vi "auxtesting_readMeasurementsCrossed.vi"() -> ()   [LabVIEW 2015, in "Tausand AB1000.lvlib"]
uses:
  <instrlib>/Tausand AB1000/Tausand AB1000.lvlib
  <instrlib>/Tausand AB1000/Public/Controls/deviceTypeRing.ctl
  <instrlib>/Tausand AB1000/Public/Controls/channelRing.ctl
panel:
  out "reading timer (s)":dbl
  out "error out":errorcluster
  in  "VISA resource name":refnum<visa-resource-name>
  in  "error in (no error)":errorcluster
  out "checksum ok?":bool
  out "read time":timestamp
  out "labels":string[](array[string])
  out "values":u32[](array[numeric])
  in  "channel":T1=1 items=["none", "A", "B", "C", "D", "E", "F", "G", "H"]
  in  "read timeout (500 ms)":u32=500
  in  "device type":T2 items=["any"=0, "AB1002"=1002, "AB1004"=1004, "AB1502"=1502, "AB1504"=1504, "AB1902"=1902, "AB1904"=1904, "AB2002"=2002, "AB2004"=2004, "AB2502"=2502, "AB2504"=2504, "AB2902"=2902, "AB2904"=2904]
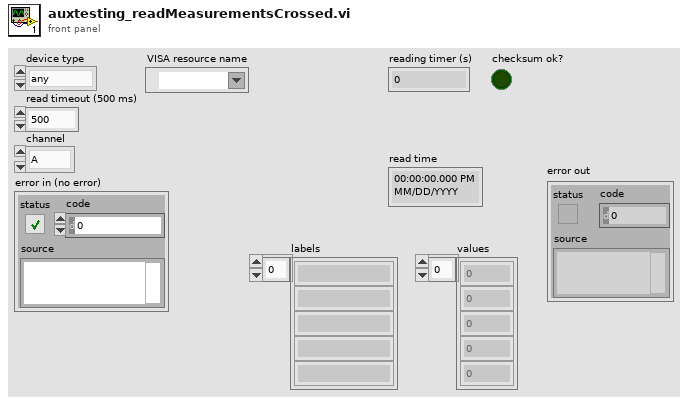
[diagram p1: front panel]
types:
  T1 = typedef "Tausand AB1000.lvlib/channelRing.ctl" = u8
  T2 = typedef "Tausand AB1000.lvlib/deviceTypeRing.ctl" = u16
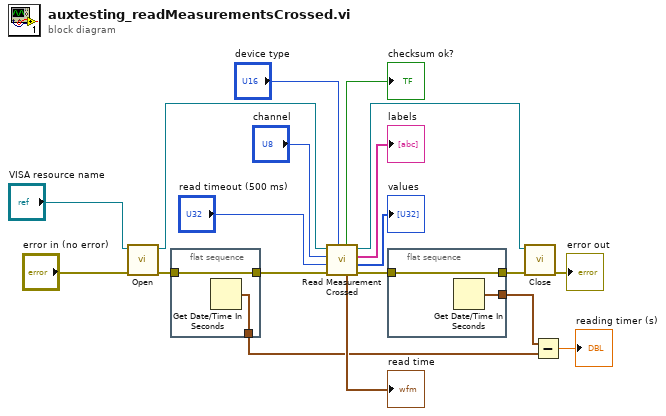
[diagram p0: block diagram]
diagram:
  n1 = call <instrlib>:"Open.vi"("error in (no error)"="error in (no error)", "VISA resource name"="VISA resource name") -> ("error out"=w6:errorcluster, "VISA resource name out"=w19:refnum<visa-resource-name>)  [unwired: 8 in]
  n2 = flat-sequence {
    tunnel: [w21] -> w7
    tunnel: w6 -> [w21]
    tunnel: [w20] -> w2
    frame #0 {
      n3 = Get Date/Time In Seconds() -> (seconds since 1Jan1904=w20:timestamp)
    }
  }
  n4 = call <instrlib>:"Read Measurement Crossed.vi"("device type"="device type", "error in (no error)"=w7, "read timeout (500 ms)"="read timeout (500 ms)", "channel"="channel", "VISA Refnum in"=w19) -> ("error out"=w5:errorcluster, "values"=→"values":u32[], "labels"=→"labels":string[], "VISA Refnum out"=w18:refnum<visa-resource-name>, "read time"=→"read time":timestamp, "checksum ok?"=→"checksum ok?":bool)  [unwired: 1 in]
  n5 = flat-sequence {
    tunnel: [w23] -> w4
    tunnel: w5 -> [w23]
    tunnel: [w22] -> w3
    frame #0 {
      n6 = Get Date/Time In Seconds() -> (seconds since 1Jan1904=w22:timestamp)
    }
  }
  n7 = call <instrlib>:"Close.vi"("error in (no error)"=w4, "VISA resource name"=w18) -> ("error out"=→"error out":errorcluster)  [unwired: 9 in]
  n8 = Subtract(x=w3, y=w2) -> (x-y=→"reading timer (s)":dbl)
